vi "Close-FpgaNic.vi"   [LabVIEW 2017]
uses:
  Globals.vi
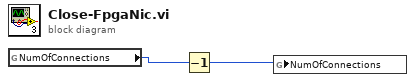
[diagram p0: block diagram]
diagram:
  n1 = global read "Globals.vi" "NumOfConnections"() -> (w2:u32)
  n2 = Decrement(x=w2) -> (x-1=w1:u32)
  n3 = global write "Globals.vi" "NumOfConnections"(w1) -> ()
